vi "SplitShiftHour.vi"(5 "BasicData":string[](array[string]), 6 "Site":i32, 8 "EndTime 2":string="12:00:00", 9 "date string":string="12/21/2014", 10 "BegTime":string="10:00:00", 11 "BegDate":string="12/20/2014") -> (3 "array":string[][](array[string]))   [LabVIEW 2012]
uses:
  <vilib>/Utility/miscctls.llb/LVDateTimeRec.ctl
  <vilib>/addons/database/Connection.llb/DB Tools Open Connec (Path).vi
  <vilib>/addons/database/Connection.llb/Conn Execute.vi
  <vilib>/addons/database/Recordset.llb/Rec Fetch Integer Data (R).vi
  <vilib>/addons/database/Recordset.llb/Rec Destroy - Connection.vi
  <vilib>/addons/database/NI_Database_API.lvlib
panel:
  out "x .and. y?":bool
  out "concatenated string":string
  out "error out":errorcluster
  in  "Cluster":T1
  out "time stamp 2":timestamp
  out "time stamp":timestamp
  in  "date time rec":T2
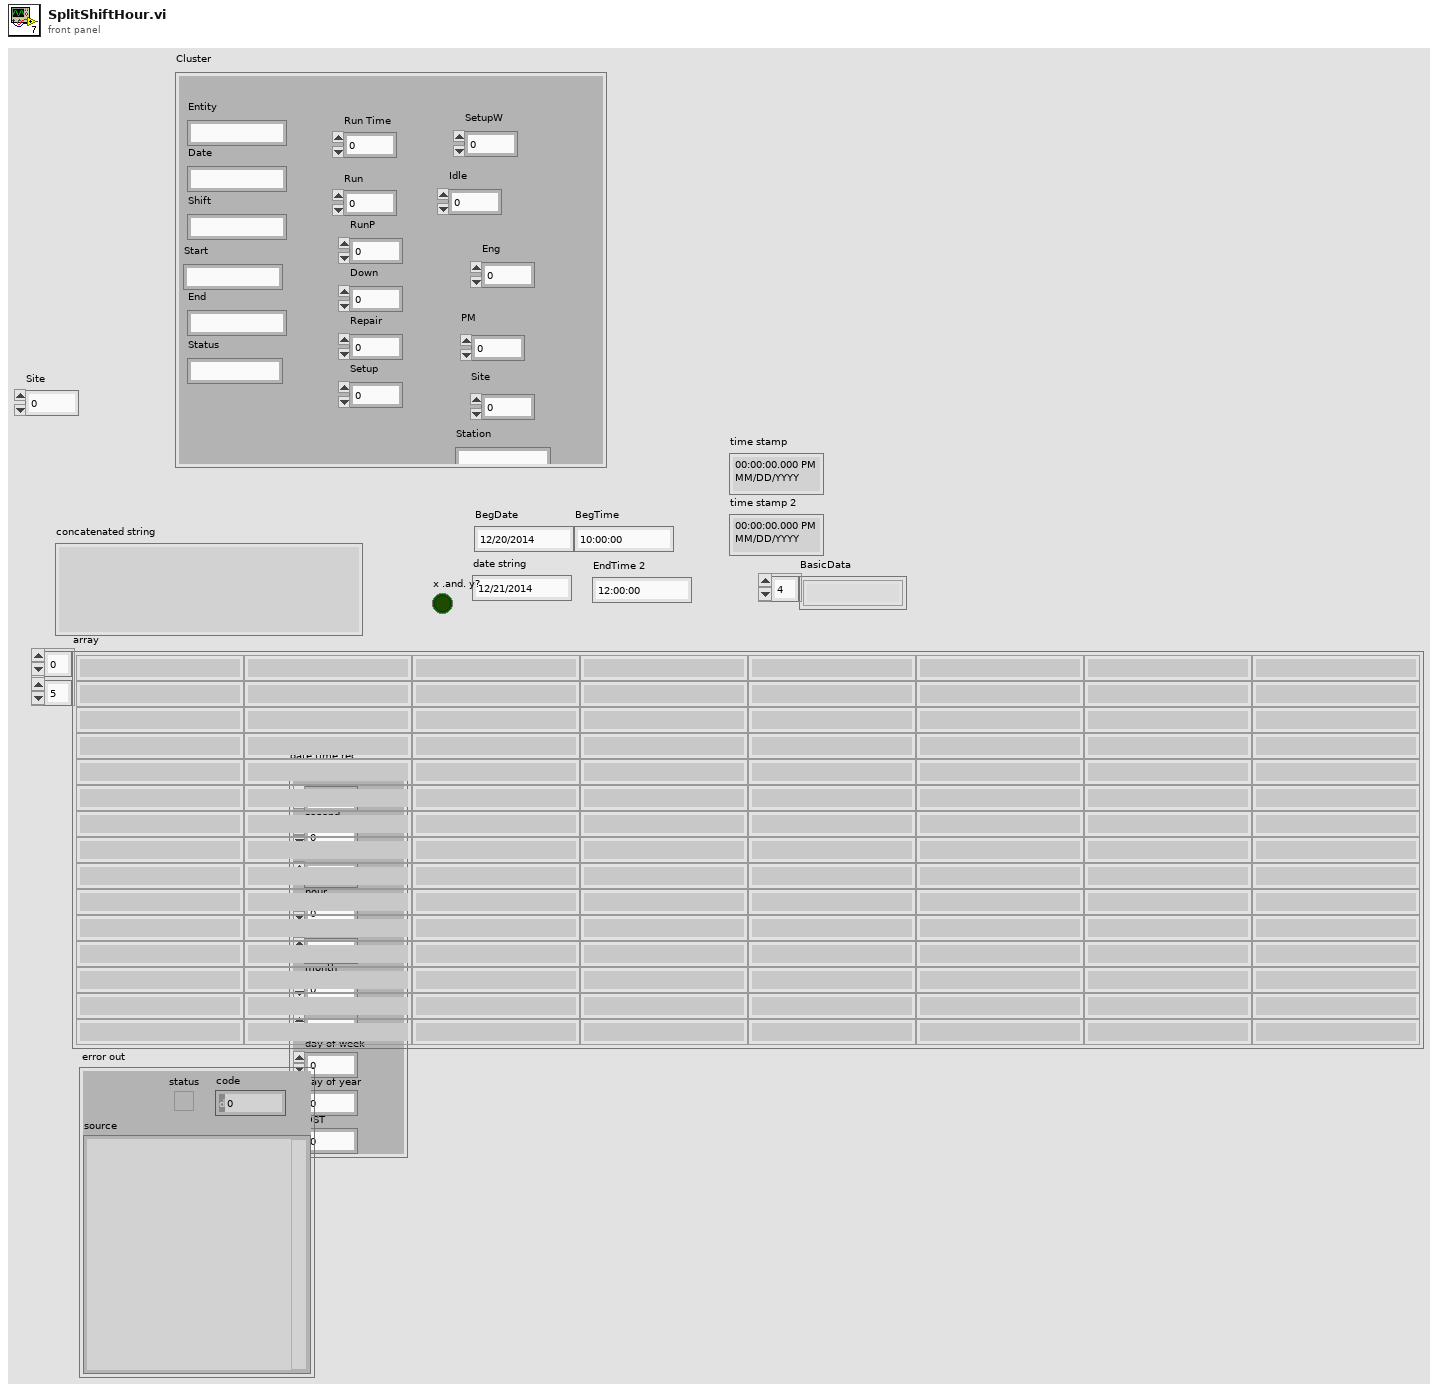
[diagram p1: front panel]
types:
  T1 = cluster{"Entity":string, "Date":string, "Shift":string, "Start":string, "End":string, "Status":string, "Run Time":dbl, "Run":dbl, "RunP":dbl, "Down":dbl, "Repair":dbl, "Setup":dbl, "SetupW":dbl, "Idle":dbl, "Eng":dbl, "PM":dbl, "Site":dbl, "Station":string}
  T2 = typedef "LVDateTimeRec.ctl" = cluster{"fractional second":dbl, "second":i32, "minute":i32, "hour":i32, "day of month":i32, "month":i32, "year":i32, "day of week":i32, "day of year":i32, "DST":i32}
  T3 = typedef "NI_Database_API.lvlib/Conn ObjectReference.ctl" = refnum<k1>
  T4 = typedef "NI_Database_API.lvlib/Rec ObjectReference.ctl" = refnum<k1>
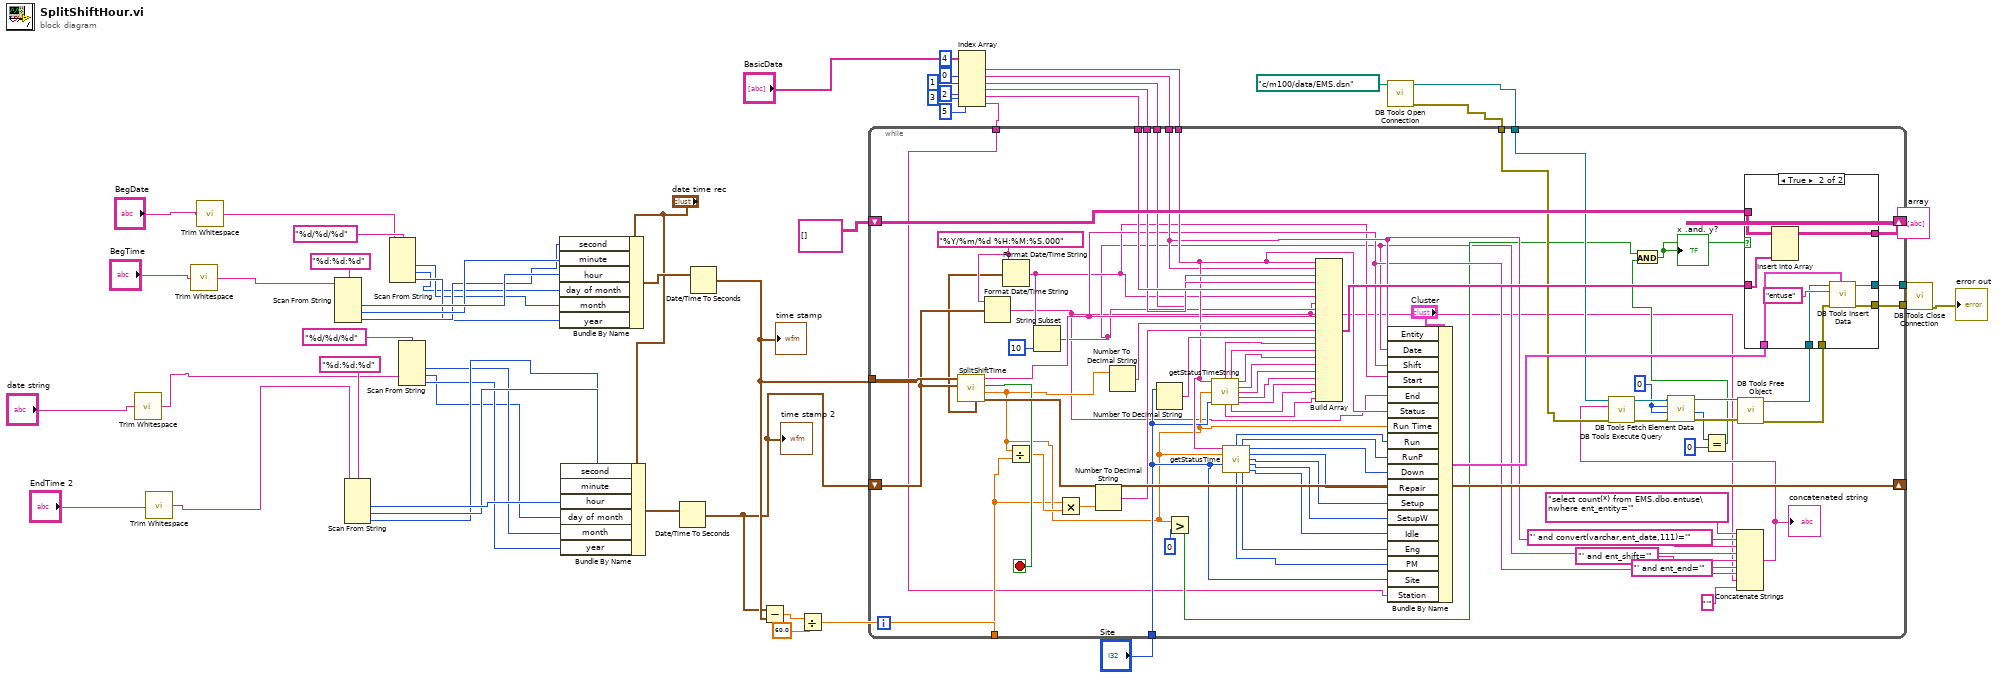
[diagram p0: block diagram]
diagram:
  n1 = call <vilib>:"Trim Whitespace.vi"("string"="date string") -> ("trimmed string"=w15:string)  [unwired: 1 in]
  n2 = call <vilib>:"Trim Whitespace.vi"("string"="EndTime 2") -> ("trimmed string"=w14:string)  [unwired: 1 in]
  n3 = call <vilib>:"Trim Whitespace.vi"("string"="BegTime") -> ("trimmed string"=w17:string)  [unwired: 1 in]
  n4 = call <vilib>:"Trim Whitespace.vi"("string"="BegDate") -> ("trimmed string"=w20:string)  [unwired: 1 in]
  n5 = Scan From String(format string="%d:%d:%d", input string=w17) -> (output 1=w52:i32, output 2=w51:i32, output 3=w50:i32)  [unwired: 5 in, 3 out]
  n6 = Scan From String(format string="%d:%d:%d", input string=w14) -> (output 1=w47:i32, output 2=w46:i32, output 3=w45:i32)  [unwired: 5 in, 3 out]
  n7 = Scan From String(format string="%d/%d/%d", input string=w20) -> (output 1=w25:i32, output 2=w24:i32, output 3=w26:i32)  [unwired: 5 in, 3 out]
  n8 = Scan From String(format string="%d/%d/%d", input string=w15) -> (output 1=w23:i32, output 2=w21:i32, output 3=w22:i32)  [unwired: 5 in, 3 out]
  n9 = Bundle By Name(cluster="date time rec", "second"=w50, "minute"=w51, "hour"=w52, "day of month"=w24, "month"=w25, "year"=w26) -> (w44:T2)
  n10 = Bundle By Name(cluster="date time rec", "second"=w45, "minute"=w46, "hour"=w47, "day of month"=w21, "month"=w23, "year"=w22) -> (w42:T2)
  n11 = Date/Time To Seconds(2:w42) -> (0:w36:timestamp)  [unwired: 1 in]
  "time stamp 2" <- w36
  n12 = Date/Time To Seconds(2:w44) -> (0:w37:timestamp)  [unwired: 1 in]
  "time stamp" <- w37
  n13 = Subtract(x=w36, y=w37) -> (x-y=w40:dbl)
  n14 = Divide(x=w40, y=60.0) -> (x/y=w38:dbl)
  n15 = Index Array(array="BasicData", index #1=4 ("index"), index #2=0 ("index"), index #3=1 ("index"), index #4=2 ("index"), index #5=3 ("index"), index #6=5 ("index")) -> (element #1=w11:string, element #2=w31:string, element #3=w32:string, element #4=w33:string, element #5=w34:string, element #6=w1:string)
  n16 = call-poly <vilib>:"DB Tools Open Connection.vi"("connection information"=path "c:/m100/data/EMS.dsn") -> ("error out"=w6:errorcluster, "connection reference"=w7:T3)  [unwired: 7 in]
  n17 = while {
    tunnel: w37 -> [w123]
    shift-right: [w125] -> _
    shift-left: w36 -> [w116]
    shift-right: [w121] -> w9
    shift-left: string[][] [] ("array") -> [w120]
    tunnel: w38 -> [w84]
    tunnel: w34 -> [w119]
    tunnel: w33 -> [w118]
    tunnel: w32 -> [w117]
    tunnel: w31 -> [w80]
    tunnel: w11 -> [w97]
    tunnel: "Site" -> [w87]
    tunnel: w7 -> [w74]
    tunnel: w6 -> [w75]
    tunnel: [w83] -> w4
    tunnel: [w82] -> w3
    tunnel: w1 -> [w55]
    stop <- w124 stop-if-true
    w66 = 0
    w114 = "%Y/%m/%d %H:%M:%S.000" ("time format string (%c)")
    n18 = call "SplitShiftTime.vi"("End"=w116, "Start"=w123) -> ("NewTime"=w125:timestamp, "Time"=w85:dbl, "ExitFlag"=w124:bool, "String"=w77:string, "start1"=w113:timestamp)  [unwired: 5 in]
    n19 = Format Date/Time String(time format string (%c)=w114, seconds (now)=w116) -> (date/time string=w57:string)  [unwired: 1 in]
    n20 = Format Date/Time String(time format string (%c)=w114, seconds (now)=w113) -> (date/time string=w60:string)  [unwired: 1 in]
    n21 = Divide(x=w85, y=w84) -> (x/y=w111:dbl)
    n22 = String Subset(string=w60, length (rest)=10 ("length (rest)")) -> (substring=w58:string)  [unwired: 1 in]
    n23 = Multiply(x=w84, y=w111) -> (x*y=w112:dbl)
    n24 = Number To Decimal String(number=w112) -> (decimal integer string=w109:string)  [unwired: 1 in]
    n25 = Number To Decimal String(number=w85) -> (decimal integer string=w115:string)  [unwired: 1 in]
    n26 = Number To Decimal String(number=w87) -> (decimal integer string=w108:string)  [unwired: 1 in]
    n27 = Greater?(x=w85, y=0) -> (0:w63:bool)
    n28 = call "getStatusTimeString.vi"("String"=w97, "Time"=w85, "Site"=w87) -> ("Run"=w107:string, "RunP"=w106:string, "Down"=w105:string, "Repair"=w104:string, "Setup"=w103:string, "SetupW"=w102:string, "PM"=w99:string, "Eng"=w100:string, "Idle"=w101:string)  [unwired: 4 in]
    n29 = call "getStatusTime.vi"("String"=w97, "Time"=w85, "Site"=w87) -> ("Run"=w96:i32, "RunP"=w95:i32, "Down"=w94:i32, "Repair"=w93:i32, "Setup"=w92:i32, "SetupW"=w91:i32, "PM"=w88:i32, "Eng"=w89:i32, "Idle"=w90:i32)  [unwired: 4 in]
    n30 = Build Array(w97, w80, w117, w118, w119, w60, w57, w58, w77, w115, w109, w108, w107, w106, w105, w104, w103, w102, w101, w100, w99) -> (w122:string[])
    n31 = Bundle By Name(cluster="Cluster", "Entity"=w80, "Date"=w58, "Shift"=w77, "Start"=w60, "End"=w57, "Status"=w97, "Run Time"=w85, "Run"=w96, "RunP"=w95, "Down"=w94, "Repair"=w93, "Setup"=w92, "SetupW"=w91, "Idle"=w90, "Eng"=w89, "PM"=w88, "Site"=w87, "Station"=w55) -> (w86:T1)
    n32 = Concatenate Strings("select count(*) from EMS.dbo.entuse\nwhere ent_entity='" ("string"), w80, "' and convert(varchar,ent_date,111)='" ("string"), w58, "' and ent_shift='" ("string"), w77, "' and ent_end='" ("string"), w57, "'" ("string")) -> (w73:string)
    "concatenated string" <- w73
    n33 = call-poly <vilib>:"DB Tools Execute Query.vi"("error in (no error)"=w75, "SQL query"=w73, "connection reference"=w74) -> ("error out"=w70:errorcluster, "recordset reference"=w72:T4)  [unwired: 5 in]
    n34 = call-poly <vilib>:"DB Tools Fetch Element Data.vi"("error in (no error)"=w70, "type"=w66, "column index"=w66, "recordset reference"=w72) -> ("error out"=w69:errorcluster, "data"=w65:i32, "recordset reference out"=w71:T4)  [unwired: 3 in]
    n35 = Equal?(x=w65, y=0) -> (x = y?=w61:bool)
    n36 = And(x=w63, y=w61) -> (x .and. y?=w62:bool)
    "x .and. y?" <- w62
    n37 = call-poly <vilib>:"DB Tools Free Object.vi"("error in (no error)"=w69, "recordset reference"=w71) -> ("error out"=w67:errorcluster, "connection reference"=w68:T3)  [unwired: 8 in]
    n38 = case shown="True" w62 {
      tunnel: w122 -> [_ w137]
      tunnel: [w128 w136] -> w121
      tunnel: w120 -> [w128 w135]
      tunnel: w86 -> [_ w133]
      tunnel: [w126 w132] -> w83
      tunnel: [w127 w131] -> w82
      tunnel: w68 -> [w126 w130]
      tunnel: w67 -> [w127 w129]
      frame False {
      }
      frame True {
        n39 = Insert Into Array(array=w135, new element=w137) -> (w136:string[][])  [unwired: 2 in]
        n40 = call <vilib>:"DB Tools Insert Data.vi"("data"=w133, "error in (no error)"=w129, "table"="entuse", "connection reference"=w130) -> ("error out"=w131:errorcluster, "connection reference out"=w132:T3)  [unwired: 6 in]
      }
    }
  }
  "array" <- w9
  n41 = call <vilib>:"DB Tools Close Connection.vi"("error in (no error)"=w3, "connection reference"=w4) -> ("error out"=→"error out":errorcluster)  [unwired: 5 in]
